vi "5668 Initiate Scan with External LO.vi"(8 "error in (no error)":errorcluster, 10 "RFSG instrument handle in":refnum<k15>, 11 "RFSA Instrument Handle In":refnum<k15>) -> (0 "error out":errorcluster, 2 "RFSG Instrument Handle Out":refnum<k15>, 3 "RFSA Instrument Handle Out":refnum<k15>)   [LabVIEW 2017]
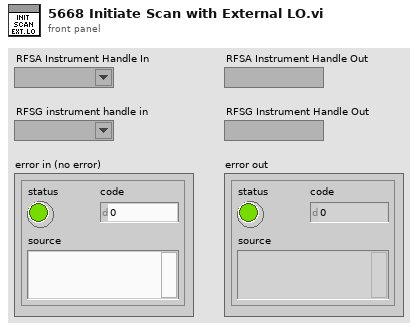
[diagram p1: front panel]
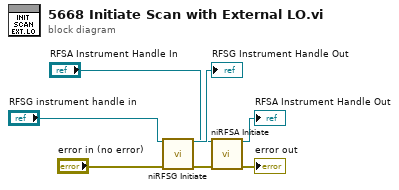
[diagram p0: block diagram]
diagram:
  n1 = call <instrlib>:"niRFSG Initiate.vi"("instrument handle"="RFSG instrument handle in", "error in"="error in (no error)") -> ("instrument handle out"=→"RFSG Instrument Handle Out":refnum<k15>, "error out"=w5:errorcluster)  [unwired: 12 in]
  n2 = call <instrlib>:"niRFSA Initiate.vi"("instrument handle"="RFSA Instrument Handle In", "error in"=w5) -> ("instrument handle out"=→"RFSA Instrument Handle Out":refnum<k15>, "error out"=→"error out":errorcluster)  [unwired: 12 in]
